vi "Post Processing.vi"() -> ()   [LabVIEW 2018]
uses:
  <vilib>/Enthought/Python Integration Toolkit/api/Console Visibility.ctl
  Global Variables.vi
  <vilib>/Enthought/Python Integration Toolkit/api/Unpack String Array.vi
  <vilib>/Enthought/Python Integration Toolkit/Python Integration Toolkit.lvlib
panel:
  out "Value":string[](array[string])
  out "XY Graph 3":cluster{dbl, "YScale.Maximum":dbl}[](graph)=[{3617058104.92992, "YScale.Maximum"=0.02}, {3617058117.2644606, "YScale.Maximum"=0.02}]
  in  "Sample Rate":i32=100
  in  "New file":bool
  in  "selected path":path=path "C:/Labview Test Data/2018-08-13/Sensors/Log_Sensors_DAQ_0.tdms"
  out "XY Graph 2":cluster{dbl, "YScale.Maximum":dbl}[](graph)=[{3617058104.92992, "YScale.Maximum"=0.02}, {3617058117.2644606, "YScale.Maximum"=0.02}]
  out "XY Graph":cluster{dbl[], dbl[]}(graph)={[3617058104.92992, 3617058105.071405, 3617058105.204719, 3617058105.339352, 3617058105.4654217, 3617058105.5895977, 3617058105.723924, 3617058105.8577886, 3617058105.9931545, 3617058106.126216, 3617058106.2686815, 3617058106.402235, 3617058106.5402184, 3617058106.6768394, 3617058106.8146977, 3617058106.9502025, 3617058107.086078, 3617058107.2211895, 3617058107.3549776, 3617058107.4918585, 3617058107.627911, 3617058107.762443, 3617058107.901148, 3617058108.034609, 3617058108.171561, 3617058108.3105903, 3617058108.448009, 3617058108.586817, 3617058108.725321, 3617058108.86412, 3617058108.9984703, 3617058109.136935, 3617058109.275936, 3617058109.415624, 3617058109.5444145, 3617058109.6839633, 3617058109.8212304, 3617058109.959656, 3617058110.099505, 3617058110.2352777, 3617058110.37625, 3617058110.5166783, 3617058110.654278, 3617058110.792069, 3617058110.9294696, 3617058111.0667214, 3617058111.2080984, 3617058111.3436384, 3617058111.4812026, 3617058111.6171255, 3617058111.754656, 3617058111.8906007, 3617058112.028036, 3617058112.1654263, 3617058112.3010263, 3617058112.437075, 3617058112.5742207, 3617058112.7098174, 3617058112.847483, 3617058112.984029, 3617058113.11964, 3617058113.256136, 3617058113.395491, 3617058113.5323257, 3617058113.6705136, 3617058113.8095255, 3617058113.945854, 3617058114.0845695, 3617058114.2227335, 3617058114.360228, 3617058114.496631, 3617058114.634196, 3617058114.77004, 3617058114.90852, 3617058115.0450034, 3617058115.1819854, 3617058115.318167, 3617058115.4536457, 3617058115.591485, 3617058115.7283754, 3617058115.870709, 3617058116.009808, 3617058116.147975, 3617058116.2889624, 3617058116.4316134, 3617058116.575004, 3617058116.7180977, 3617058116.860796, 3617058117.000852, 3617058117.1353416, 3617058117.2644606], array[9200 elements]}
  out "Selected Channel":u32=2
  in  "stop":bool
  in  "Array":string[](array[string])=["Current_0", "Current_1", "Current_2", "Current_3", "Current_4", "Current_5", "Current_6", "Current_7"]
  in  "Cut":bool
  in  "Final Time":timestamp=timestamp(3617058117.2644606 s since 1904-01-01) format="%<%X\n%x>T"
  in  "Inital Time":timestamp=timestamp(3617058104.92992 s since 1904-01-01) format="%<%X\n%x>T"
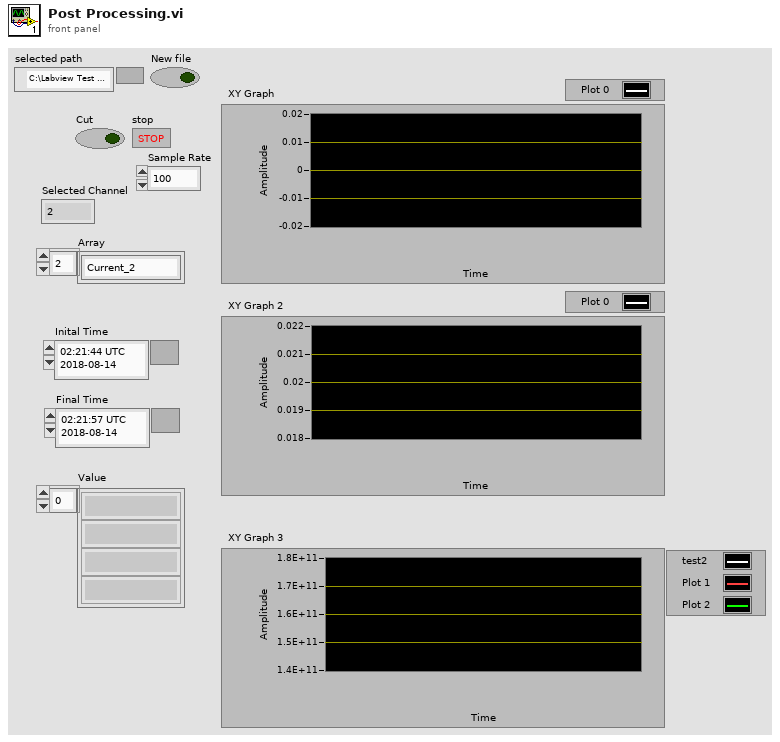
[diagram p1: front panel]
types:
  T1 = typedef "Python Integration Toolkit.lvlib/Console Visibility.ctl" = enum16{"Show Console", "Show Console While Running", "Hide Console"}
  T2 = enum16{"open", "open or create", "create or replace", "create", "open (read-only)"}
  T3 = typedef "Python Integration Toolkit.lvlib/Session ID.ctl" = u64
  T4 = typedef "Python Integration Toolkit.lvlib/Python Objects.ctl" = variant
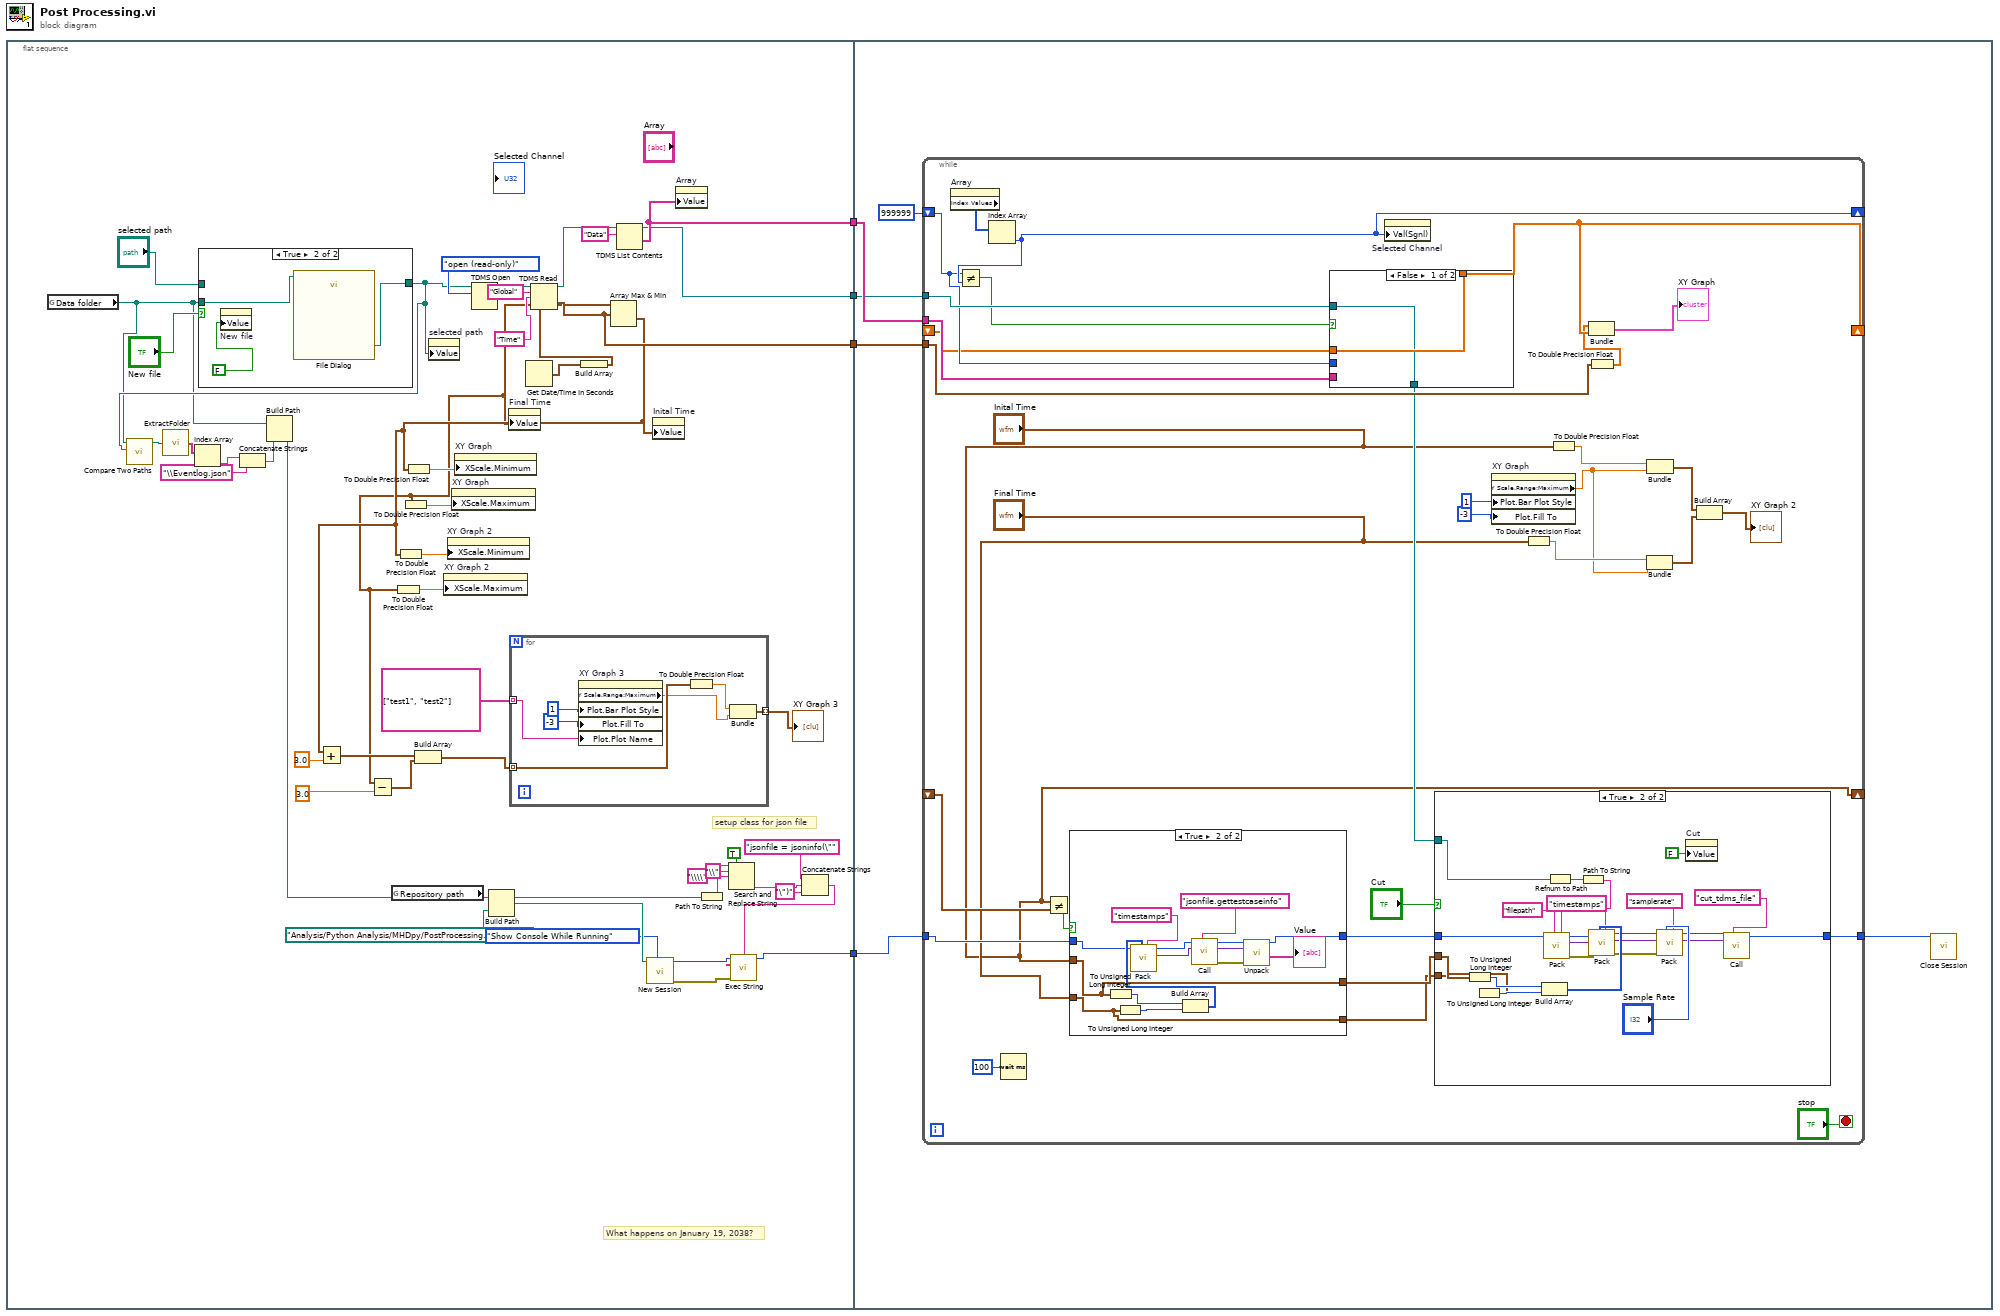
[diagram p0: block diagram]
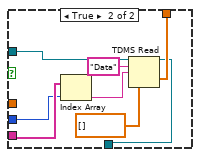
[diagram p5: hidden frame]
diagram:
  n1 = flat-sequence {
    tunnel: [w45] -> w4
    tunnel: [w43] -> w3
    tunnel: [w44] -> w2
    tunnel: [w10] -> w1
    tunnel: w4 -> [w70]
    tunnel: w3 -> [w69]
    tunnel: w2 -> [w68]
    tunnel: w1 -> [w66]
    frame #0 {
      # "setup class for json file"
      # "What happens on January 19, 2038?"
      n2 = global read "Global Variables.vi" "Data folder"() -> (w21:path)
      n3 = case shown="True" "New file" {
        tunnel: [w61 w64] -> w23
        tunnel: "selected path" -> [w61 _]
        tunnel: w21 -> [_ w62]
        frame False {
        }
        frame True {
          n4 = property on="New file" class="Bool (strict)"("Value"=FALSE ("New file")) -> ()  [unwired: 2 in, 2 out]
          n5 = call "File Dialog"("start path"=w62) -> ("selected path"=w64:path)  [unwired: 11 in, 3 out]
        }
      }
      n6 = call <vilib>:"Compare Two Paths.vi"("Path 2"=w23, "Path 1"=w21) -> ("Relative Path from 1 to 2"=w22:path)  [unwired: 6 in, 3 out]
      n7 = call "ExtractFolder.vi"("path"=w22) -> ("Array"=w20:string[])
      n8 = Index Array(array=w20) -> (element=w19:string)  [unwired: 1 in]
      n9 = Concatenate Strings(w19, "\\Eventlog.json" ("string")) -> (w17:string)
      n10 = Build Path(base path=w21, name or relative path=w17) -> (appended path=w16:path)
      n11 = global read "Global Variables.vi" "Repository path"() -> (w38:path)
      n12 = property on="selected path" class="Path"("Value"=w23) -> ()  [unwired: 2 in, 2 out]
      n13 = TDMS Open(10:T2."open (read-only)" ("operation (0:open)"), 11:w23) -> (3:w52:refnum<k34>)  [unwired: 5 in, 1 out]
      n14 = Build Path(base path=w38, name or relative path=path "Analysis/Python Analysis/MHDpy/PostProcessing.py" ("Repository path")) -> (appended path=w36:path)
      n15 = Get Date/Time In Seconds() -> (seconds since 1Jan1904=w49:timestamp)
      n16 = Build Array(w49) -> (w48:timestamp[])
      n17 = TDMS Read(0:w52, 5:"Global" ("group name in"), 7:"Time" ("group name in"), 12:w48) -> (4:w47:refnum<k34>, 10:w43:timestamp[])  [unwired: 4 in, 4 out]
      n18 = Array Max & Min(array=w43) -> (max value=w26:timestamp, min value=w29:timestamp)  [unwired: 2 out]
      n19 = Add(x=w29, y=3.0) -> (x+y=w28:timestamp)
      n20 = Subtract(x=w26, y=3.0) -> (x-y=w24:timestamp)
      n21 = To Double Precision Float(number=w26) -> (double precision float=w40:dbl)
      n22 = To Double Precision Float(number=w29) -> (double precision float=w39:dbl)
      n23 = To Double Precision Float(number=w26) -> (double precision float=w41:dbl)
      n24 = To Double Precision Float(number=w29) -> (double precision float=w42:dbl)
      n25 = Build Array(w28, w24) -> (w31:timestamp[])
      n26 = property on="XY Graph 2" class="XYGraph (strict)"("XScale.Maximum"=w40) -> ()  [unwired: 2 in, 2 out]
      n27 = property on="XY Graph 2" class="XYGraph (strict)"("XScale.Minimum"=w39) -> ()  [unwired: 2 in, 2 out]
      n28 = property on="XY Graph" class="XYGraph (strict)"("XScale.Maximum"=w41) -> ()  [unwired: 2 in, 2 out]
      n29 = property on="XY Graph" class="XYGraph (strict)"("XScale.Minimum"=w42) -> ()  [unwired: 2 in, 2 out]
      n30 = property on="Final Time" class="AbsTime (strict)"("Value"=w26) -> ()  [unwired: 2 in, 2 out]
      n31 = for {
        tunnel: string[] ["test1", "test2"] -> [w56] mode=indexing
        tunnel: w31 -> [w58] mode=indexing
        tunnel: [w57] -> w30 mode=indexing
        n32 = property on="XY Graph 3" class="XYGraph (strict)"("Plot.Bar Plot Style"=u8 1, "Plot.Fill To"=i16 -3, "Plot.Plot Name"=w56) -> ("Y Scale.Range:Maximum"=w55:dbl)  [unwired: 2 in, 2 out]
        n33 = To Double Precision Float(number=w58) -> (double precision float=w54:dbl)
        n34 = Bundle(w54, "YScale.Maximum"=w55) -> (w57:cluster{dbl, "YScale.Maximum":dbl})  [unwired: 1 in]
      }
      "XY Graph 3" <- w30
      n35 = TDMS List Contents(6:"Data" ("group name"), 7:w47) -> (1:w45:string[], 3:w44:refnum<k34>)  [unwired: 1 in, 2 out]
      n36 = call <vilib>:"New Session.vi"("Console Visibility"=Console_Visibility."Show Console While Running", "Path to Python Module (.py File)"=w36) -> ("error out"=w12:errorcluster, "Session ID out"=w13:T3)  [unwired: 8 in]
      n37 = property on="Inital Time" class="AbsTime (strict)"("Value"=w29) -> ()  [unwired: 2 in, 2 out]
      n38 = property on="Array" class="Arr (strict)"("Value"=w45) -> ()  [unwired: 2 in, 2 out]
      n39 = Path To String(path=w16) -> (string=w9:string)
      n40 = Search and Replace String(replace all?=TRUE ("replace all? (F)"), input string=w9, search string="\\", replace string="\\\\" ("replace string (\"\")")) -> (result string=w6:string)  [unwired: 4 in, 3 out]
      n41 = Concatenate Strings("jsonfile = jsoninfo(\"" ("string"), w6, "\")" ("string")) -> (w11:string)
      n42 = call <vilib>:"Exec String.vi"("error in (no error)"=w12, "Python Code"=w11, "Session ID"=w13) -> ("Session ID out"=w10:T3)  [unwired: 7 in, 1 out]
    }
    frame #1 {
      n43 = while {
        tunnel: w69 -> [w93]
        tunnel: w68 -> [w98]
        tunnel: w70 -> [w99]
        shift-right: [w92] -> _
        shift-left: _ -> [w94]
        shift-right: [w97] -> _
        shift-left: u32 999999 -> [w95]
        tunnel: w66 -> [w76]
        tunnel: [w80] -> w65
        shift-right: ["Inital Time"] -> _
        shift-left: _ -> [w78]
        stop <- "stop" stop-if-true
        n44 = property on="Array" class="Arr (strict)"() -> ("Index Values"=w100:u32[])  [unwired: 2 in, 2 out]
        n45 = Index Array(array=w100) -> (element=w97:u32)  [unwired: 1 in]
        n46 = Not Equal?(x=w95, y=w97) -> (x != y?=w96:bool)
        n47 = Wait (ms)(milliseconds to wait=u32 100) -> ()  [unwired: 1 out]
        n48 = Not Equal?(x="Inital Time", y=w78) -> (x != y?=w77:bool)
        n49 = case shown="True" w77 {
          tunnel: w76 -> [w105 w115]
          tunnel: [w105 w107] -> w75
          tunnel: "Final Time" -> [w103 w112]
          tunnel: "Inital Time" -> [w104 w113]
          tunnel: [w104 w113] -> w72
          tunnel: [w103 w112] -> w71
          frame False {
          }
          frame True {
            n50 = To Unsigned Long Integer(number=w113) -> (unsigned 32bit integer=w117:u32)
            n51 = To Unsigned Long Integer(number=w112) -> (unsigned 32bit integer=w118:u32)
            n52 = Build Array(w117, w118) -> (w116:u32[])
            n53 = call <vilib>:"Pack.vi"("Keyword Name"="timestamps" ("Function or Method Name"), "Argument"=w116, "Session ID"=w115) -> ("Python Object References Out"=w111:T4, "Session ID out"=w114:T3)  [unwired: 6 in, 1 out]
            n54 = call <vilib>:"Call.vi"("Function or Method Name"="jsonfile.gettestcaseinfo", "Python Object References In"=w111, "Session ID"=w114) -> ("error out"=w110:errorcluster, "Python Object References Out"=w109:T4, "Session ID out"=w108:T3)  [unwired: 6 in]
            n55 = call-poly <vilib>:"Unpack.vi"("error in (no error)"=w110, "Python Object References In"=w109, "Session ID"=w108) -> ("Value"=→"Value":string[], "Session ID out"=w107:T3)  [unwired: 5 in, 2 out]
          }
        }
        n56 = case shown="False" w96 {
          tunnel: w99 -> [_ w155]
          tunnel: w98 -> [w146 w154]
          tunnel: [w147 w153] -> w92
          tunnel: w95 -> [_ w150]
          tunnel: w94 -> [w147 _]
          tunnel: [w146 w148] -> w81
          frame False {
          }
          frame True {
            n57 = Index Array(array=w155, index=w150) -> (element=w151:string)
            n58 = TDMS Read(0:w154, 5:"Data" ("group name in"), 7:w151, 12:dbl[] []) -> (4:w148:refnum<k34>, 10:w153:dbl[])  [unwired: 4 in, 4 out]
          }
        }
        n59 = property on="Selected Channel" class="DigNum (strict)"("Val(Sgnl)"=w97) -> ()  [unwired: 2 in, 2 out]
        n60 = case shown="True" "Cut" {
          tunnel: w72 -> [_ w123]
          tunnel: w71 -> [_ w122]
          tunnel: w75 -> [w121 w143]
          tunnel: w81 -> [_ w145]
          tunnel: [w121 w142] -> w80
          frame False {
          }
          frame True {
            n61 = To Unsigned Long Integer(number=w123) -> (unsigned 32bit integer=w125:u32)
            n62 = To Unsigned Long Integer(number=w122) -> (unsigned 32bit integer=w124:u32)
            n63 = Build Array(w125, w124) -> (w137:u32[])
            n64 = Refnum to Path(1:w145) -> (0:w144:path)
            n65 = Path To String(path=w144) -> (string=w136:string)
            n66 = call <vilib>:"Pack.vi"("Keyword Name"="filepath", "Argument"=w136, "Session ID"=w143) -> ("error out"=w140:errorcluster, "Python Object References Out"=w139:T4, "Session ID out"=w138:T3)  [unwired: 6 in]
            n67 = call <vilib>:"Pack.vi"("Keyword Name"="timestamps", "Argument"=w137, "error in (no error)"=w140, "Python Object References In"=w139, "Session ID"=w138) -> ("error out"=w132:errorcluster, "Python Object References Out"=w131:T4, "Session ID out"=w130:T3)  [unwired: 4 in]
            n68 = call <vilib>:"Pack.vi"("Keyword Name"="samplerate", "Argument"="Sample Rate", "error in (no error)"=w132, "Python Object References In"=w131, "Session ID"=w130) -> ("Python Object References Out"=w126:T4, "Session ID out"=w127:T3)  [unwired: 4 in, 1 out]
            n69 = property on="Cut" class="Bool (strict)"("Value"=FALSE ("Cut")) -> ()  [unwired: 2 in, 2 out]
            n70 = call <vilib>:"Call.vi"("Function or Method Name"="cut_tdms_file" ("Keyword Name"), "Python Object References In"=w126, "Session ID"=w127) -> ("Session ID out"=w142:T3)  [unwired: 6 in, 2 out]
          }
        }
        n71 = property on="XY Graph" class="XYGraph (strict)"("Plot.Bar Plot Style"=u8 1, "Plot.Fill To"=i16 -3) -> ("Y Scale.Range:Maximum"=w82:dbl)  [unwired: 2 in, 2 out]
        n72 = To Double Precision Float(number="Final Time") -> (double precision float=w87:dbl)
        n73 = To Double Precision Float(number="Inital Time") -> (double precision float=w88:dbl)
        n74 = To Double Precision Float(number=w93) -> (double precision float=w91:dbl[])
        n75 = Bundle(w91, w92) -> (→"XY Graph":cluster{dbl[], dbl[]})  [unwired: 1 in]
        n76 = Bundle(w87, "YScale.Maximum"=w82) -> (w84:cluster{dbl, "YScale.Maximum":dbl})  [unwired: 1 in]
        n77 = Bundle(w88, "YScale.Maximum"=w82) -> (w85:cluster{dbl, "YScale.Maximum":dbl})  [unwired: 1 in]
        n78 = Build Array(w85, w84) -> (→"XY Graph 2":cluster{dbl, "YScale.Maximum":dbl}[])
      }
      n79 = call <vilib>:"Close Session.vi"("Session ID"=w65) -> ()  [unwired: 10 in, 1 out]
    }
  }
